vi "process.vi"(8 "error in":errorcluster, 9 "result allocation":T1, 10 "parameters":T1, 11 "module in":refnum<class "Multiplexer runtime.lvclass">) -> (0 "error out":errorcluster, 1 "results":T1, 2 "parameter allocation":T1, 3 "module out":refnum<class "Multiplexer runtime.lvclass">)   [LabVIEW 2021, in "Multiplexer runtime.lvclass"]
doc: "Provides an interface for information processing by a module at runtime. While this interface performs no operations, a child should provide an override which may process data in any manner necessary."
uses:
  Multiplexer runtime.lvclass
  <vilib>/NI/Tag Bus/table/data table.ctl
  Multiplexer runtime.lvclass/Multiplexer runtime.ctl
  <vilib>/NI/Tag Bus/table/data polymorphs/read many/read Doubles.vi
  <vilib>/NI/Tag Bus/table/data polymorphs/read one/read Boolean.vi
  <vilib>/NI/Tag Bus/table/data polymorphs/write one/write Double.vi
  <vilib>/NI/Tag Bus/table/data table.lvlib
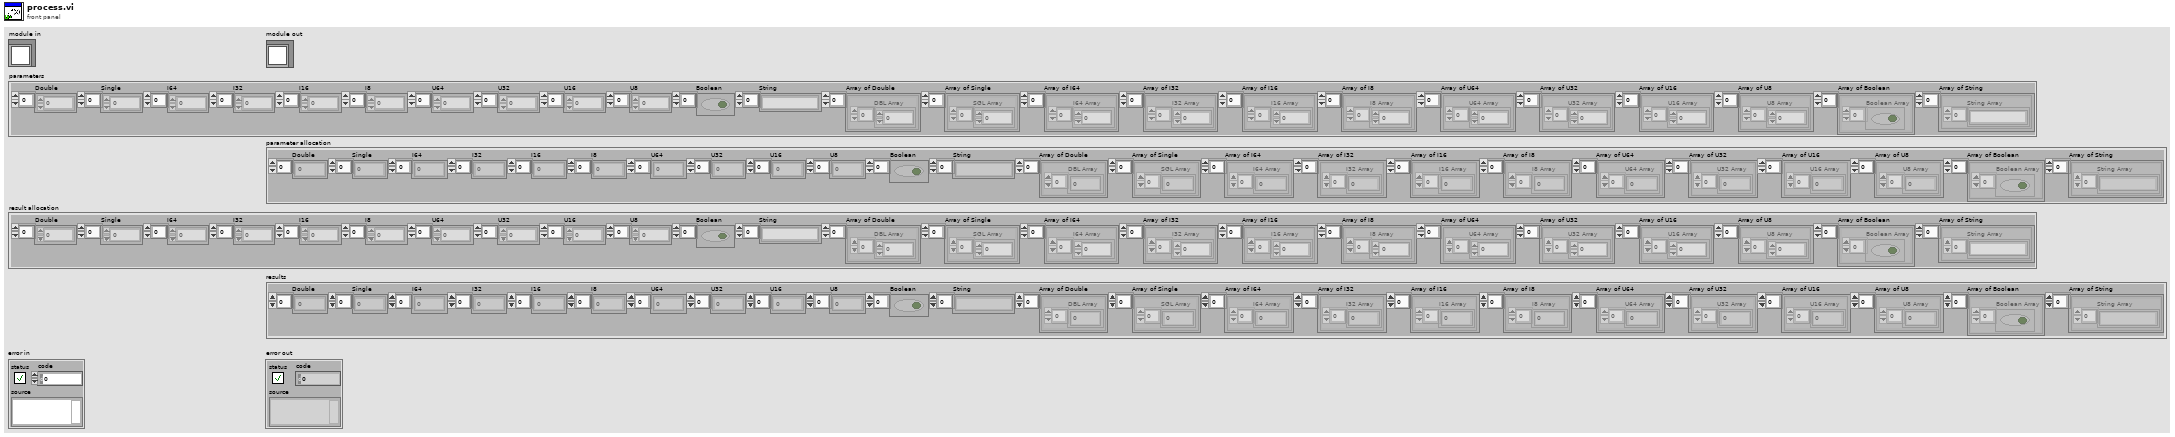
[diagram p1: front panel]
types:
  T1 = typedef "tag bus.lvlib/data table.lvlib/data table.ctl" = cluster{"Double":dbl[], "Single":sgl[], "I64":i64[], "I32":i32[], "I16":i16[], "I8":i8[], "U64":u64[], "U32":u32[], "U16":u16[], "U8":u8[], "Boolean":bool[], "String":string[], "Array of Double":cluster{"DBL Array":dbl[]}[], "Array of Single":cluster{"SGL Array":sgl[]}[], "Array of I64":cluster{"I64 Array":i64[]}[], "Array of I32":cluster{"I32 Array":i32[]}[], "Array of I16":cluster{"I16 Array":i16[]}[], "Array of I8":cluster{"I8 Array":i8[]}[], "Array of U64":cluster{"U64 Array":u64[]}[], "Array of U32":cluster{"U32 Array":u32[]}[], "Array of U16":cluster{"U16 Array":u16[]}[], "Array of U8":cluster{"U8 Array":u8[]}[], "Array of Boolean":cluster{"Boolean Array":bool[]}[], "Array of String":cluster{"String Array":string[]}[]}
  T2 = typedef "Multiplexer runtime.lvclass/Line Mappings.ctl" = cluster{"A":i32, "B":i32, "Select":i32, "Output":i32}
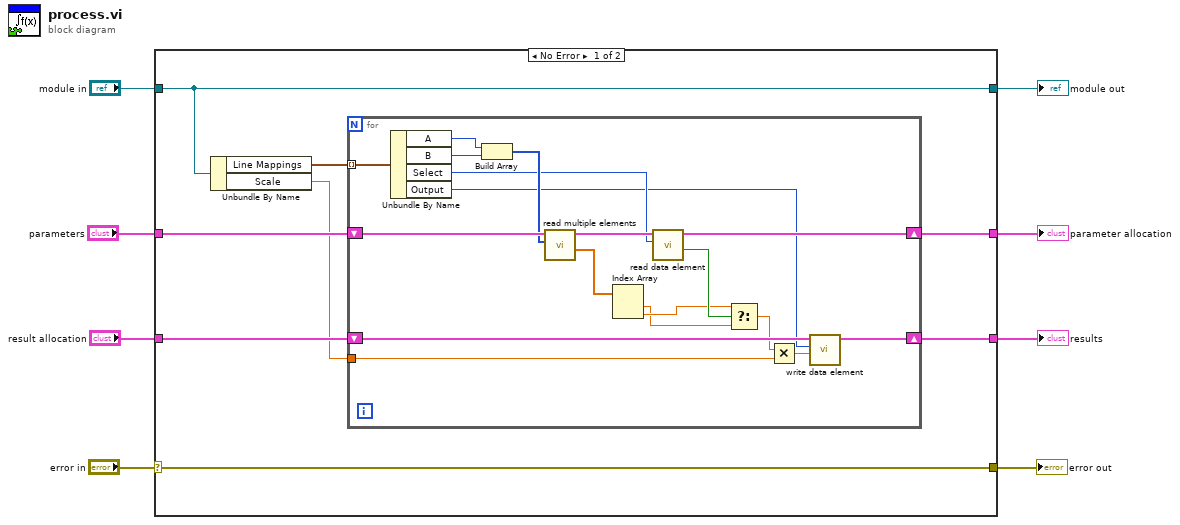
[diagram p0: block diagram]
diagram:
  n1 = case shown="No Error" "error in" {
    selector: "error in" -> [w16 w38]
    tunnel: [w16 w38] -> w7
    tunnel: [w13 w37] -> w5
    tunnel: "module in" -> [w13 w37]
    tunnel: "parameters" -> [w15 w36]
    tunnel: "result allocation" -> [w14 w35]
    tunnel: [w10 w36] -> w2
    tunnel: [w9 w35] -> w1
    frame No Error {
      n2 = Unbundle By Name(w13) -> ("Line Mappings"=w12:T2[], "Scale"=w11:dbl)
      n3 = for {
        shift-right: [w28] -> w10
        shift-left: w15 -> [w31]
        shift-right: [w25] -> w9
        shift-left: w14 -> [w26]
        tunnel: w12 -> [w34] mode=indexing
        tunnel: w11 -> [w19]
        n4 = Unbundle By Name(w34) -> ("A"=w33:i32, "B"=w32:i32, "Select"=w27:i32, "Output"=w24:i32)
        n5 = Build Array(w33, w32) -> (w30:i32[])
        n6 = call-poly <vilib>:"read multiple elements.vi"("indices"=w30, "data table in"=w31) -> ("values"=w23:dbl[], "data table out"=w29:T1)  [unwired: 8 in]
        n7 = Index Array(array=w23) -> (element #1=w17:dbl, element #2=w18:dbl)  [unwired: 2 in]
        n8 = call-poly <vilib>:"read data element.vi"("index"=w27, "data table in"=w29) -> ("value"=w22:bool, "data table out"=w28:T1)  [unwired: 8 in]
        n9 = Select(t=w18, s=w22, f=w17) -> (s? t:f=w20:dbl)
        n10 = Multiply(x=w20, y=w19) -> (x*y=w21:dbl)
        n11 = call-poly <vilib>:"write data element.vi"("value"=w21, "index"=w24, "data table in"=w26) -> ("data table out"=w25:T1)  [unwired: 8 in]
      }
    }
    frame Error {
    }
  }
  "error out" <- w7
  "module out" <- w5
  "results" <- w1
  "parameter allocation" <- w2
